vi "Retriggerable_Finite_Counter_20230330.vi"() -> ()   [LabVIEW 2021]
uses:
  <resource>/objmgr/daqmx.rc
  <vilib>/Utility/error.llb/DialogType.ctl
  <vilib>/DAQmx/configure/timing.llb/DAQmx Timing (Sample Clock).vi
  <vilib>/DAQmx/create/channels.llb/DAQmx Create Channel (CI-Count Edges).vi
  <vilib>/DAQmx/read.llb/DAQmx Read (Counter 1D U32 1Chan NSamp).vi
  <vilib>/DAQmx/configure/timing.llb/DAQmx Timing (Implicit).vi
  <vilib>/DAQmx/create/channels.llb/DAQmx Create Channel (CO-Pulse Generation-Frequency).vi
  <vilib>/DAQmx/configure/events/hardwareSignals.llb/DAQmx Export Signal (Most Signals).vi
  <vilib>/DAQmx/read.llb/DAQmx Read (Analog 1D Wfm NChan NSamp).vi
  <vilib>/DAQmx/create/channels.llb/DAQmx Create Channel (AI-Voltage-Basic).vi
  <vilib>/DAQmx/write.llb/DAQmx Write (Analog DBL 1Chan 1Samp).vi
panel:
  in  "AI Physical Channel":tag="Dev2/ai0"
  out "Read Iteration.":i32=20 caption="Read Iteration.\nIf working correctly,\nthis should increment\nonce per second."
  out "Actual Duty Cycle":dbl=0.01
  out "Actual Frequency":dbl=1.0
  in  "Duty Cycle":dbl=0.01 caption="Duty Cycle Must Be Less Than Sampling Duration (%)" format="%.6f"
  in  "Frequency (Hz)":dbl=1.0 format="%.6f"
  in  "Output Terminal":tag="/Dev2/PFI12" caption="Output Terminal For Routing to First Counter"
  in  "Counter 2":tag="Dev2/ctr1"
  out "Total Count\nThis is the":u32 caption="Total Count.\nThis is what you're most interested in."
  in  "Stop":bool
  in  "Trigger Type":enum32{"No Trigger", "Digital Arm Start"}(tab)=enum."Digital Arm Start"
  in  "Edge":i32(ring)=10280 items=["Rising"=10280, "Falling"=10171]
  out "Data":u32[](array[numeric])
  in  "Samples":i32=1000
  in  "Signal Input Terminal":tag="PFI8"
  in  "Counter":tag="Dev2/ctr0"
  in  "Sample Rate":dbl=100000.0
  in  "Sample Clock Source":tag="/Dev2/PFI14"
  # "Task 1: Finite Counter Measurement"
  # "Task 2: Create Sample Clock"
  # "Task 2: Create Slow Pulse Train"
  # "Lots of count values. (You can delete this indicator.\nI've left it here to make it easier to understand how this is working.)"
  # "To configure and use a trigger or the count reset you must have the \"Digital Arm Start\"  tab selected."
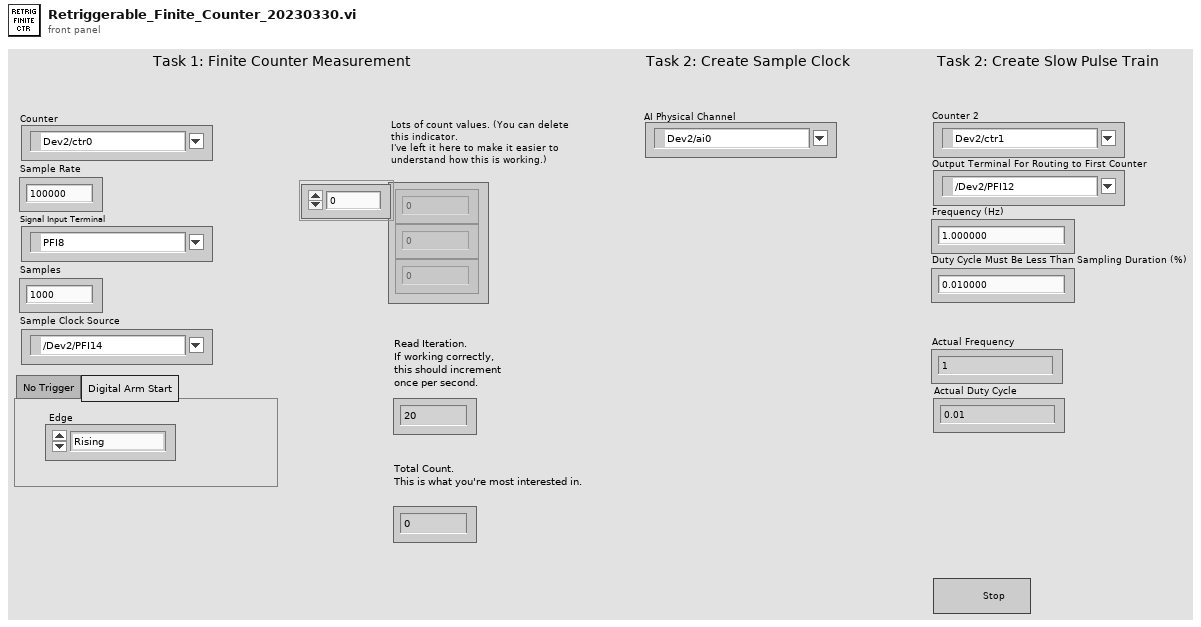
[diagram p1: front panel]
types:
  T1 = typedef "DialogType.ctl" = u16
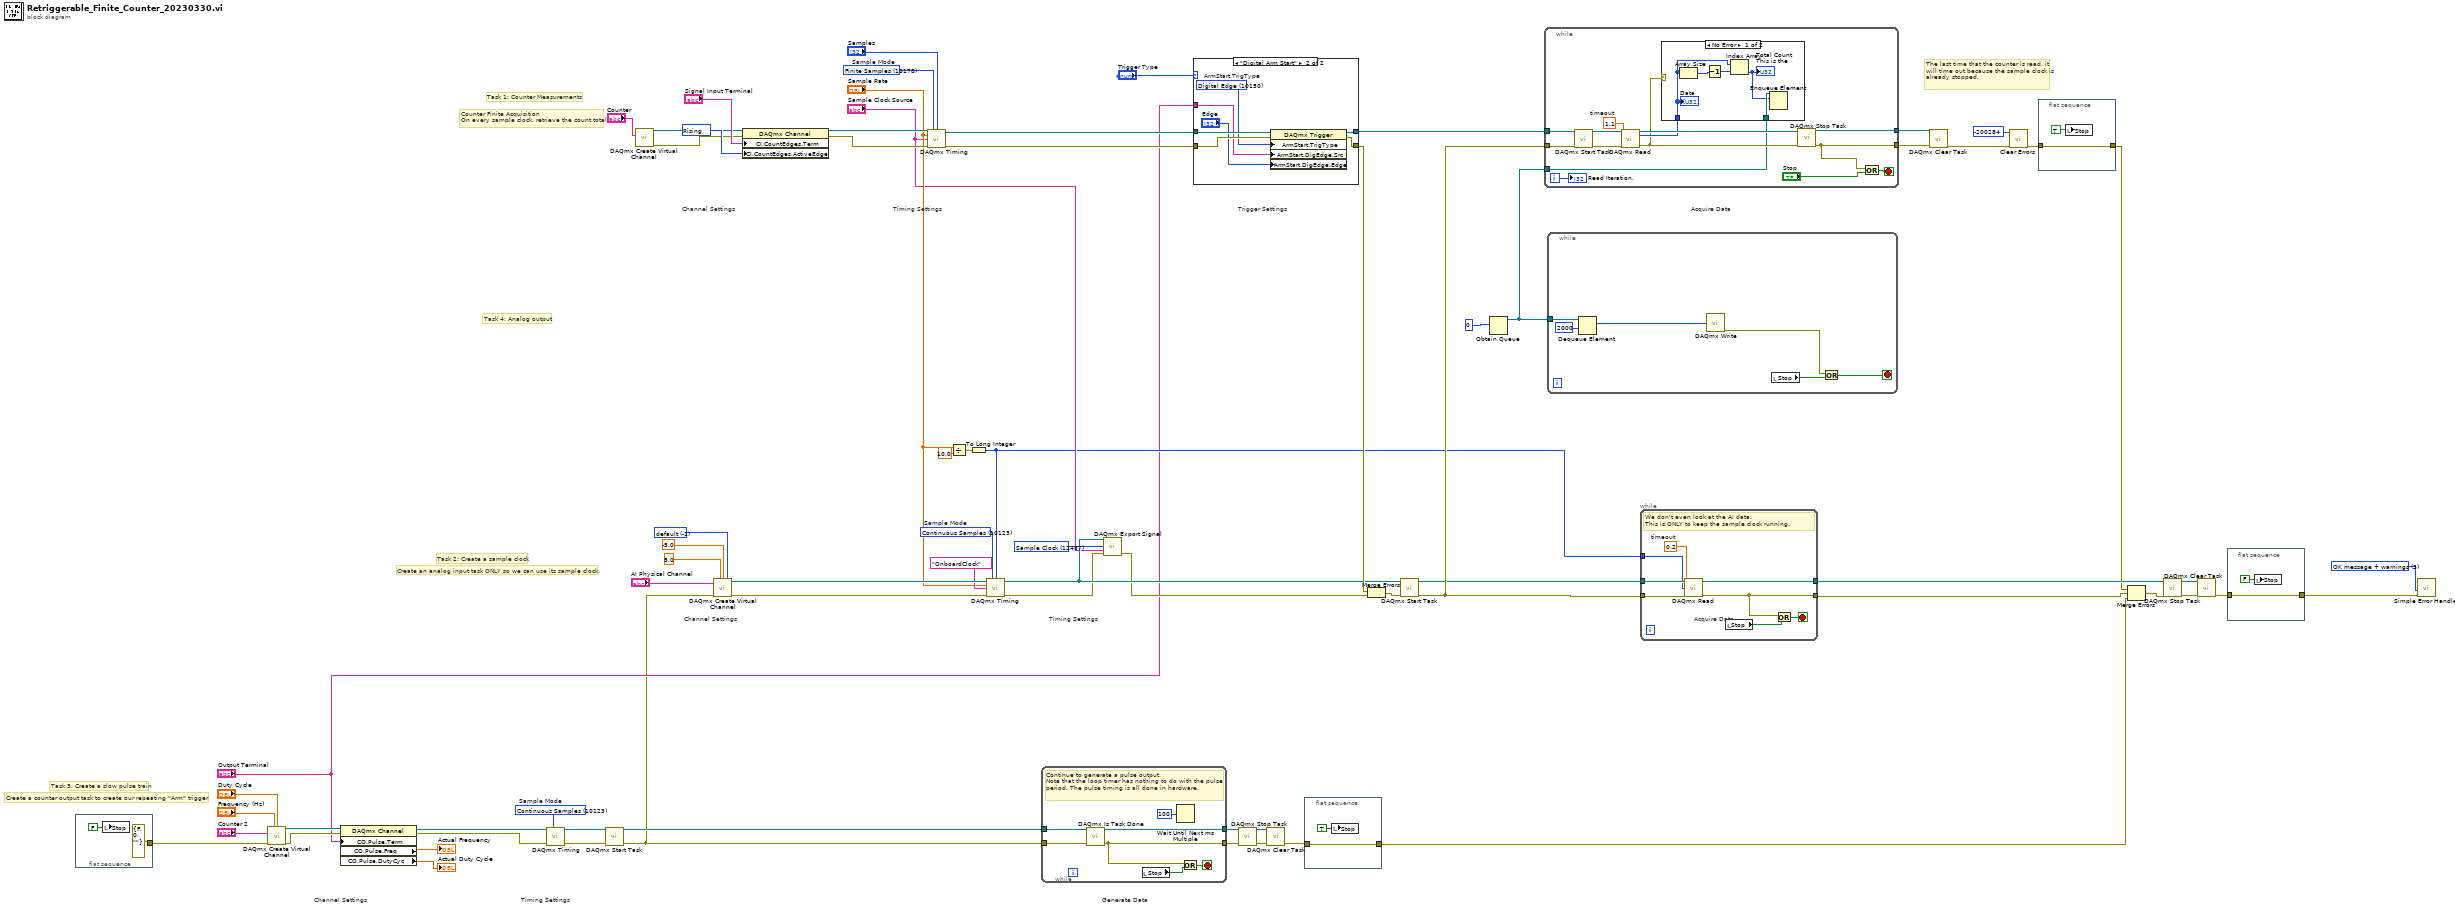
[diagram p0: block diagram]
diagram:
  w71 = 10280 items=["Rising"=10280, "Falling"=10171] ("Active Edge")
  w29 = 10123 items=["Finite Samples"=10178, "Continuous Samples"=10123, "Hardware Timed Single Point"=12522]  # Sample Mode
  w35 = 12487 items=["AI Convert Clock"=12484, "10MHz Reference Clock"=12536, "20MHz Timebase Clock"=12486, "Sample Clock"=12487, "Advance Trigger"=12488, "Reference Trigger"=12490, "Start Trigger"=12491, "Advance Complete Event"=12492, "AI Hold Complete Event"=12493, "Counter Output Event"=12494, "Change Detection Event"=12511, "Watchdog Timer Expired Event"=12512] ("signal")
  w55 = -1 items=["default"=-1, "RSE"=10083, "NRSE"=10078, "Differential"=10106, "Pseudodifferential"=12529] ("Terminal Configuration")
  w48 = T1 3 items=["no dialog", "OK message", "continue or stop message", "OK message + warnings", "continue/stop + warnings"] ("type of dialog (OK msg:1)")
  w59 = 10123 items=["Finite Samples"=10178, "Continuous Samples"=10123, "Hardware Timed Single Point"=12522]  # Sample Mode
  w70 = 10178 items=["Finite Samples"=10178, "Continuous Samples"=10123, "Hardware Timed Single Point"=12522]  # Sample Mode
  # "Task 4: Analog output"
  # "Task 3: Create a slow pulse train"
  # "Task 2: Create a sample clock"
  # "Task 1: Counter Measurements"
  # "The last time that the counter is read, it will time out because the sample clock is already stopped."
  # "Create a counter output task to create our repeating \"Arm\" trigger"
  # "Generate Data"
  # "Timing Settings"
  # "Channel Settings"
  # "Create an analog input task ONLY so we can use its sample clock."
  # "Counter Finite Acquisition\nOn every sample clock, retrieve the count total"
  # "Acquire Data"
  # "Timing Settings"
  # "Channel Settings"
  # "Acquire Data"
  # "Trigger Settings"
  # "Timing Settings"
  # "Channel Settings"
  n1 = flat-sequence {
    tunnel: [errorcluster {"status"=FALSE, "code"=0, "source"=""} ("error out")] -> w8
    frame #0 {
      n2 = local write "Stop"(FALSE ("Stop")) -> ()
    }
  }
  n3 = call-poly <vilib>:"DAQmx Create Virtual Channel.vi"("frequency"="Frequency (Hz)", "duty cycle"="Duty Cycle", "counter"="Counter 2", "error in"=w8) -> ("task out"=w24:refnum<k21>, "error out"=w23:errorcluster)  [unwired: 10 in]
  n4 = property class="DAQmx Channel"(reference=w24, error in=w23, "CO.Pulse.Term"="Output Terminal") -> (reference out=w21:refnum<k21>, error out=w22:errorcluster, "CO.Pulse.Freq"=→"Actual Frequency":dbl, "CO.Pulse.DutyCyc"=→"Actual Duty Cycle":dbl)
  n5 = call-poly <vilib>:"DAQmx Timing.vi"("task/channels in"=w21, "sample mode"=w29, "error in"=w22) -> ("task out"=w26:refnum<k21>, "error out"=w25:errorcluster)  [unwired: 11 in]
  n6 = call <vilib>:"DAQmx Start Task.vi"("task/channels in"=w26, "error in"=w25) -> ("task out"=w28:refnum<k21>, "error out"=w9:errorcluster)  [unwired: 12 in]
  n7 = call-poly <vilib>:"DAQmx Create Virtual Channel.vi"("counter"="Counter") -> ("task out"=w68:refnum<k21>, "error out"=w65:errorcluster)  [unwired: 13 in]
  n8 = call-poly <vilib>:"DAQmx Create Virtual Channel.vi"("maximum value"=5.0 ("Max Voltage"), "minimum value"=-5.0 ("Min Voltage"), "input terminal configuration"=w55, "physical channels"="AI Physical Channel", "error in"=w9) -> ("task out"=w57:refnum<k21>, "error out"=w58:errorcluster)  [unwired: 9 in]
  n9 = property class="DAQmx Channel"(reference=w68, error in=w65, "CI.CountEdges.Term"="Signal Input Terminal", "CI.CountEdges.ActiveEdge"=w71) -> (reference out=w67:refnum<k21>, error out=w66:errorcluster)
  n10 = call-poly <vilib>:"DAQmx Timing.vi"("task/channels in"=w67, "sample mode"=w70, "samples per channel"="Samples", "rate"="Sample Rate", "source"="Sample Clock Source", "error in"=w66) -> ("task out"=w61:refnum<k21>, "error out"=w62:errorcluster)  [unwired: 8 in]
  n11 = Divide(x="Sample Rate", y=10.0) -> (x/y=w39:dbl)
  n12 = To Long Integer(number=w39) -> (32bit integer=w32:i32)
  n13 = call-poly <vilib>:"DAQmx Timing.vi"("task/channels in"=w57, "sample mode"=w59, "samples per channel"=w32, "rate"="Sample Rate", "source"=tag "OnboardClock" ("Sample Clock Source 2"), "error in"=w58) -> ("task out"=w38:refnum<k21>, "error out"=w37:errorcluster)  [unwired: 8 in]
  n14 = while {
    tunnel: w28 -> [w81]
    tunnel: w9 -> [w80]
    tunnel: [w77] -> w13
    tunnel: [w78] -> w14
    stop <- w79 stop-if-true
    # "Continue to generate a pulse output. \nNote that the loop timer has nothing to do with the pulse period. The pulse timing is all done in hardware."
    n15 = call <vilib>:"DAQmx Is Task Done.vi"("task/channels in"=w81, "error in"=w80) -> ("task out"=w78:refnum<k21>, "error out"=w77:errorcluster)  [unwired: 11 in, 1 out]
    n16 = local read "Stop"() -> (w75:bool)
    n17 = Wait Until Next ms Multiple(millisecond multiple=u32 100) -> ()  [unwired: 1 out]
    n18 = Or(x=w77, y=w75) -> (x .or. y?=w79:bool)
  }
  n19 = call-poly <vilib>:"DAQmx Export Signal.vi"("task/channels in"=w38, "signal"=w35, "output terminal"="Sample Clock Source", "error in"=w37) -> ("error out"=w36:errorcluster)  [unwired: 10 in, 1 out]
  n20 = case shown="\"Digital Arm Start\"" "Trigger Type" {
    tunnel: w61 -> [w83 w90]
    tunnel: w62 -> [w82 w87]
    tunnel: [w83 w89] -> w60
    tunnel: [w82 w88] -> w46
    tunnel: "Output Terminal" -> [_ w84]
    frame "No Trigger", Default {
    }
    frame "Digital Arm Start" {
      w85 = 10150 items=["Digital Edge"=10150, "None"=10230]  # ArmStart.TrigType
      n21 = property class="DAQmx Trigger"(reference=w90, error in=w87, "ArmStart.TrigType"=w85, "ArmStart.DigEdge.Src"=w84, "ArmStart.DigEdge.Edge"="Edge") -> (reference out=w89:refnum<k21>, error out=w88:errorcluster)
    }
  }
  n22 = call <vilib>:"DAQmx Stop Task.vi"("task/channels in"=w14, "error in"=w13) -> ("task out"=w16:refnum<k21>, "error out"=w15:errorcluster)  [unwired: 12 in]
  n23 = call <vilib>:"DAQmx Clear Task.vi"("task in"=w16, "error in"=w15) -> ("error out"=w11:errorcluster)  [unwired: 13 in]
  n24 = flat-sequence {
    tunnel: [w91] -> w10
    tunnel: w11 -> [w91]
    frame #0 {
      n25 = local write "Stop"(TRUE ("Stop")) -> ()
    }
  }
  n26 = Merge Errors(w46, w36) -> (w47:errorcluster)
  n27 = call <vilib>:"DAQmx Start Task.vi"("task/channels in"=w38, "error in"=w47) -> ("task out"=w33:refnum<k21>, "error out"=w45:errorcluster)  [unwired: 12 in]
  n28 = Obtain Queue(element data type=u32 0 ("Total Count\nThis is the 2")) -> (queue out=w2:refnum<queue>)  [unwired: 4 in, 2 out]
  n29 = while {
    tunnel: w60 -> [w104]
    tunnel: [w98] -> w7
    tunnel: [w97] -> w6
    tunnel: w45 -> [w102]
    tunnel: w2 -> [w94]
    i -> [w99]
    stop <- w100 stop-if-true
    w96 = 1.1  # timeout
    n30 = call <vilib>:"DAQmx Start Task.vi"("task/channels in"=w104, "error in"=w102) -> ("task out"=w106:refnum<k21>, "error out"=w105:errorcluster)  [unwired: 12 in]
    n31 = call-poly <vilib>:"DAQmx Read.vi"("task/channels in"=w106, "timeout"=w96, "error in"=w105) -> ("task out"=w103:refnum<k21>, "data"=w101:u32[], "error out"=w95:errorcluster)  [unwired: 10 in]
    n32 = case shown="No Error" w95 {
      tunnel: w101 -> [w109 _]
      tunnel: w94 -> [w108 _]
      frame No Error {
        n33 = Array Size(array=w109) -> (size(s)=w111:i32)
        n34 = Decrement(x=w111) -> (x-1=w110:i32)
        n35 = Index Array(array=w109, index=w110) -> (element=w107:u32)
        "Total Count\nThis is the" <- w107
        n36 = Enqueue Element(queue=w108, element=w107) -> ()  [unwired: 2 in, 3 out]
        "Data" <- w109
      }
      frame Error {
      }
    }
    n37 = call <vilib>:"DAQmx Stop Task.vi"("task/channels in"=w103, "error in"=w95) -> ("task out"=w98:refnum<k21>, "error out"=w97:errorcluster)  [unwired: 12 in]
    n38 = Or(x=w97, y="Stop") -> (x .or. y?=w100:bool)
    "Read Iteration." <- w99
  }
  n39 = while {
    tunnel: w2 -> [w117]
    stop <- w113 stop-if-true
    n40 = Dequeue Element(queue=w117, timeout in ms (-1)=2000) -> (element=w116:u32)  [unwired: 1 in, 3 out]
    n41 = call-poly <vilib>:"DAQmx Write.vi"("data"=w116) -> ("error out"=w114:errorcluster)  [unwired: 12 in, 2 out]
    n42 = local read "Stop"() -> (w115:bool)
    n43 = Or(x=w114, y=w115) -> (x .or. y?=w113:bool)
  }
  n44 = while {
    tunnel: w33 -> [w125]
    tunnel: w45 -> [w124]
    tunnel: [w123] -> w51
    tunnel: [w122] -> w44
    tunnel: w32 -> [w120]
    stop <- w121 stop-if-true
    w119 = 0.2  # timeout
    # "We don't even look at the AI data.\nThis is ONLY to keep the sample clock running."
    n45 = call-poly <vilib>:"DAQmx Read.vi"("task/channels in"=w125, "number of samples per channel"=w120, "timeout"=w119, "error in"=w124) -> ("task out"=w123:refnum<k21>, "error out"=w122:errorcluster)  [unwired: 9 in, 1 out]
    n46 = local read "Stop"() -> (w118:bool)
    n47 = Or(x=w122, y=w118) -> (x .or. y?=w121:bool)
  }
  n48 = call <vilib>:"DAQmx Clear Task.vi"("task in"=w7, "error in"=w6) -> ("error out"=w5:errorcluster)  [unwired: 13 in]
  n49 = call <vilib>:"Clear Errors.vi"("error in (no error)"=w5, "specific error code to clear (0: all)"=-200284) -> ("error out"=w4:errorcluster)  [unwired: 4 in, 1 out]
  n50 = flat-sequence {
    tunnel: [w126] -> w42
    tunnel: w4 -> [w126]
    frame #0 {
      n51 = local write "Stop"(TRUE ("Stop")) -> ()
    }
  }
  n52 = Merge Errors(w42, w44, w10) -> (w43:errorcluster)
  n53 = call <vilib>:"DAQmx Stop Task.vi"("task/channels in"=w51, "error in"=w43) -> ("task out"=w49:refnum<k21>, "error out"=w50:errorcluster)  [unwired: 12 in]
  n54 = call <vilib>:"DAQmx Clear Task.vi"("task in"=w49, "error in"=w50) -> ("error out"=w31:errorcluster)  [unwired: 13 in]
  n55 = flat-sequence {
    tunnel: [w128] -> w30
    tunnel: w31 -> [w128]
    frame #0 {
      n56 = local write "Stop"(FALSE ("Stop")) -> ()
    }
  }
  n57 = call <vilib>:"Simple Error Handler.vi"("type of dialog (OK msg:1)"=w48, "error in (no error)"=w30) -> ()  [unwired: 3 in, 5 out]
